vi "niFPGA Shift 4 Saturate (to I32).vi"(2 "I32 input":i32 format="%08x") -> (6 "saturated I32 output":i32 format="%.0x")   [LabVIEW 2017]
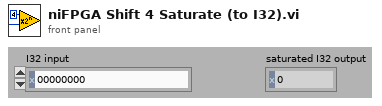
[diagram p1: front panel]
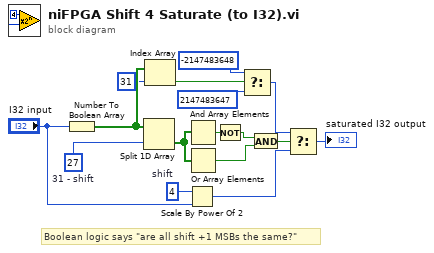
[diagram p0: block diagram]
diagram:
  w16 = i8 4  # shift
  w15 = i8 27  # 31 - shift
  # "Boolean logic says \"are all shift +1 MSBs the same?\""
  n1 = Number To Boolean Array(number="I32 input") -> (Boolean array=w12:bool[])
  n2 = Split 1D Array(array=w12, index=w15) -> (second subarray=w13:bool[])  [unwired: 1 out]
  n3 = Index Array(array=w12, index=31) -> (element=w10:bool)
  n4 = Scale By Power Of 2(n=w16, x="I32 input") -> (x*2^n=w1:i32)
  n5 = And Array Elements(Boolean array=w13) -> (logical AND=w6:bool)
  n6 = Or Array Elements(Boolean array=w13) -> (logical OR=w4:bool)
  n7 = Not(x=w6) -> (.not. x?=w5:bool)
  n8 = Select(t=-2147483648, s=w10, f=2147483647) -> (s? t:f=w2:i32)
  n9 = And(x=w5, y=w4) -> (x .and. y?=w3:bool)
  n10 = Select(t=w2, s=w3, f=w1) -> (s? t:f=→"saturated I32 output":i32)
